vi "Test Case No Error.vi"() -> ()   [LabVIEW 2015]
uses:
  JSONtext.lvlib
panel:
  out "Test Cases results 2":string[](array[string])
  out "Should be Error":errorcluster[](array[cluster])
  out "Should be no Error":errorcluster[](array[cluster])
  out "Test Cases results":string[](array[string])
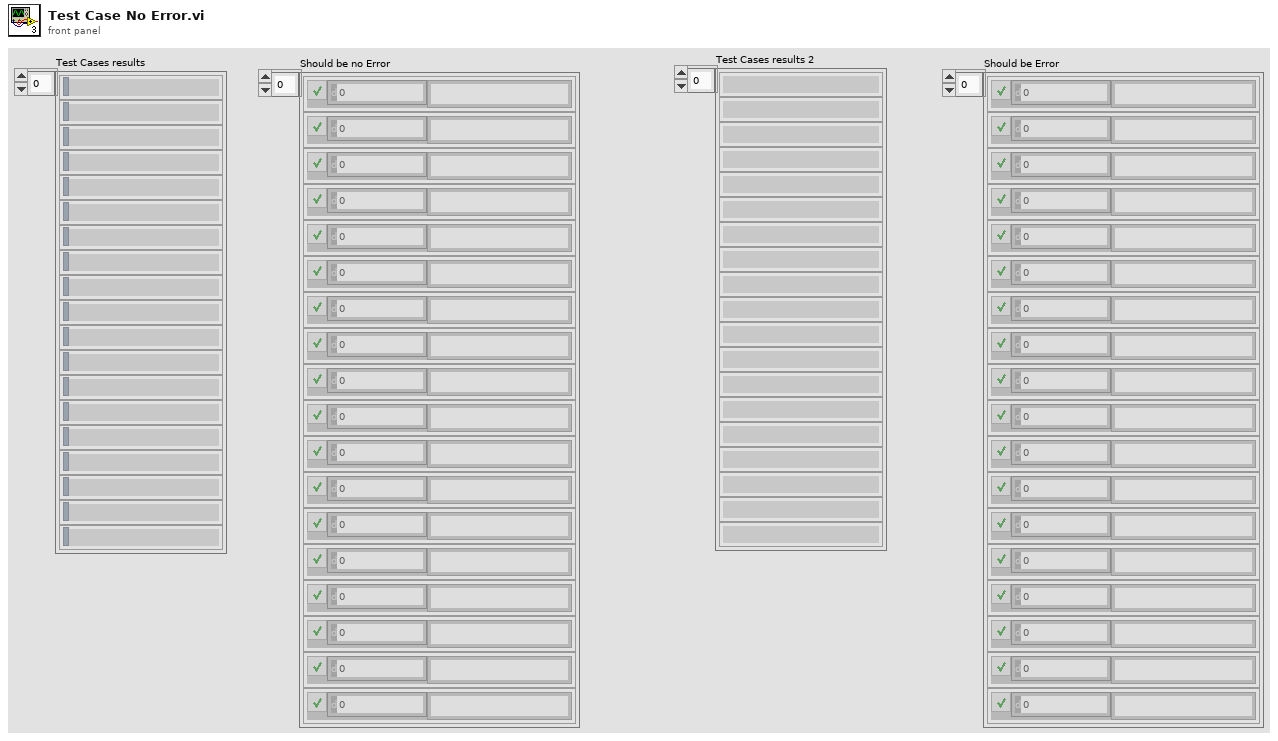
[diagram p1: front panel]
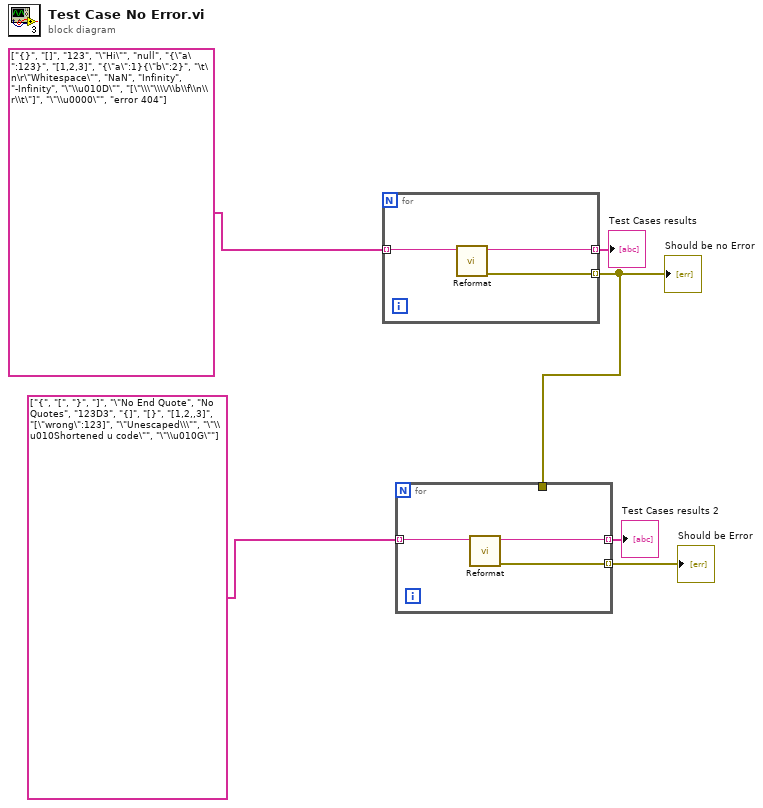
[diagram p0: block diagram]
diagram:
  n1 = for {
    tunnel: string[] ["{}", "[]", "123", "\"Hi\"", "null", "{\"a\":123}", "[1,2,3]", "{\"a\":1}{\"b\":2}", "\t\n\r\"Whitespace\"", "NaN", "Infinity", "-Infinity", "\"\\u010D\"", "[\"\\\"\\\\/\\b\\f\\n\\r\\t\"]", "\"\\u0000\"", "error 404"] -> [w9] mode=indexing
    tunnel: [w8] -> w5 mode=indexing
    tunnel: [w7] -> w1 mode=indexing
    n2 = call "Reformat.vi"("Input String"=w9) -> ("error out"=w7:errorcluster, "<JSON>First JSON Value"=w8:string)  [unwired: 7 in, 2 out]
  }
  "Test Cases results" <- w5
  "Should be no Error" <- w1
  n3 = for {
    tunnel: string[] ["{", "[", "}", "]", "\"No End Quote", "No Quotes", "123D3", "{]", "[}", "[1,2,,3]", "[\"wrong\":123]", "\"Unescaped\\\"", "\"\\u010Shortened u code\"", "\"\\u010G\""] -> [w12] mode=indexing
    tunnel: [w11] -> w3 mode=indexing
    tunnel: [w10] -> w4 mode=indexing
    tunnel: w1 -> [_]
    n4 = call "Reformat.vi"("Input String"=w12) -> ("error out"=w10:errorcluster, "<JSON>First JSON Value"=w11:string)  [unwired: 7 in, 2 out]
  }
  "Test Cases results 2" <- w3
  "Should be Error" <- w4
